vi "Catcher.vi"(0 "Catcher Position":i8) -> ()   [LabVIEW 2012]
uses:
  Robot Global Data.vi
  <vilib>/Rock Robotics/WPI/Joystick/WPI_JoystickGetSetRefNum.vi
panel:
  in  "Roller Speed Hold Low":dbl=-0.3
  out "High-Speed Toggle":bool
  in  "Bridge Position":dbl=2.8
  out "Joystick Control":bool
  in  "Joystick Speed Divider":dbl=2.0
  in  "Joystick Up Factor":dbl=1.5
  in  "Roller Speed Hold High":dbl=-0.3
  out "Button 11 Toggle":bool
  in  "Perimeter Threshold":dbl=1.1
  in  "Max Speeds":cluster{"Down Speed":dbl, "Up Speed":dbl}={"Down Speed"=0.45, "Up Speed"=-0.7}
  in  "PID gains":T1={"proportional gain (Kc)"=1.0, "integral time (Ti, min)"=0.0, "derivative time (Td, min)"=0.0} {"derivative time (Td, min)" format="%.3f"; "integral time (Ti, min)" format="%.3f"; "proportional gain (Kc)" format="%.3f"}
  out "Override":bool
  in  "Roller Speed Shoot":dbl=0.4
  in  "Dump Position":dbl=3.5
  out "Inside Perimeter":bool=TRUE
  in  "Catch Position":dbl=4.5
  in  "Rest Position":dbl=1.0
  out "Pot Voltage":dbl=1.0584093950000002
  # "0 - Hold Position\n1 - Catch\n2 - Dump\n4 - Bridge\n8 - Rest"
  # "4.5"
  # "0.8"
  # "0.35"
  # "3.5"
  # "-0.45"
  # "-0.6"
  # "2.8"
  # "-0.5"
  # "1"
  # "0.85"
  # "1"
  # "0"
  # "0"
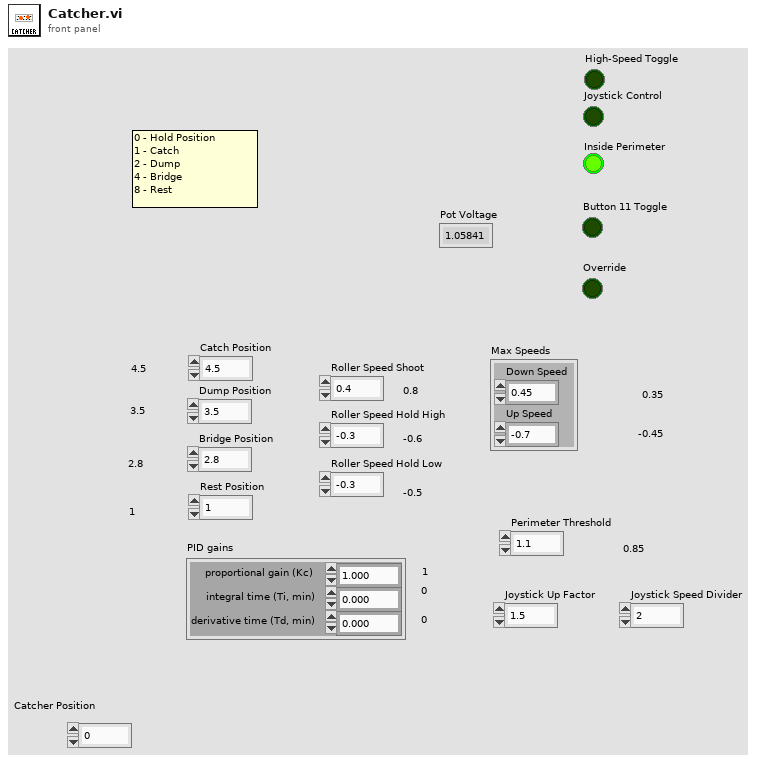
[diagram p1: front panel]
types:
  T1 = cluster{"proportional gain (Kc)":dbl, "integral time (Ti, min)":dbl, "derivative time (Td, min)":dbl}
  T2 = typedef "WPI_JoystickDevRef.ctl" = cluster{"Device":T3}
  T3 = typedef "WPI_JoystickDeviceEnum.ctl" = enum16{"USB 1", "USB 2", "USB 3", "USB 4", "Kinect 1", "Kinect 2"}
  T4 = typedef "WPI_JoystickButtonState.ctl" = cluster{"Button 1":bool, "Button 2":bool, "Button 3":bool, "Button 4":bool, "Button 5":bool, "Button 6":bool, "Button 7":bool, "Button 8":bool, "Button 9":bool, "Button 10":bool, "Button 11":bool, "Button 12":bool}
  T5 = cluster{"axis 1 (x)":dbl, "axis 2 (y)":dbl, "axis 3 (throttle)":dbl, "axis 4":dbl, "axis 5":dbl, "axis 6":dbl}
  T6 = typedef "WPI_AnalogChannelDevRef.ctl" = cluster{"DevStatus":errorcluster, "Analog Module":T7, "Analog Channel":T8}
  T7 = typedef "FPGA_TypedefAnalogModule.ctl" = enum16{"Analog Module 1", "Analog Module 2"}
  T8 = typedef "FPGA_AIChannel.ctl" = enum8{"AI 1", "AI 2", "AI 3", "AI 4", "AI 5", "AI 6", "AI 7", "AI 8", "Invalid"}
  T9 = typedef "WPI_MotorControlDeviceRef.ctl" = cluster{"DeviceStatus":errorcluster, "Type":enum16{"PWM", "CAN"}, "PWM":cluster{"Digital Module":T10, "PWM Channel":T11, "DeadBand":T12}, "CAN":cluster{"Device Number":u8, "Control Mode":T13, "Semaphore":T14, "Max Vout":dbl}, "Invert":bool, "TransformRef":T15, "InvTransformRef":T15}
  T10 = typedef "FPGA_TypedefDigitalModule.ctl" = enum16{"Digital Module 1", "Digital Module 2"}
  T11 = typedef "FPGA_DIOPWMChannel.ctl" = enum8{"PWM 1", "PWM 2", "PWM 3", "PWM 4", "PWM 5", "PWM 6", "PWM 7", "PWM 8", "PWM 9", "PWM 10", "Invalid"}
  T12 = typedef "WPI_PWMDeadband.ctl" = cluster{"Name":string, "maxPositivePwm":i32, "minPositivePwm":i32, "centerPwm":i32, "maxNegativePwm":i32, "minNegativePwm":i32, "angularRange":u16}
  T13 = typedef "WPI_CANJaguar_ControlMode.ctl" = enum8{"Percent VBus", "Current", "Speed", "Position", "Voltage"}
  T14 = typedef "Semaphore RefNum" = refnum<k1>
  T15 = typedef "WPI_PWMTransform_ConPane.ctl" = refnum<vi>
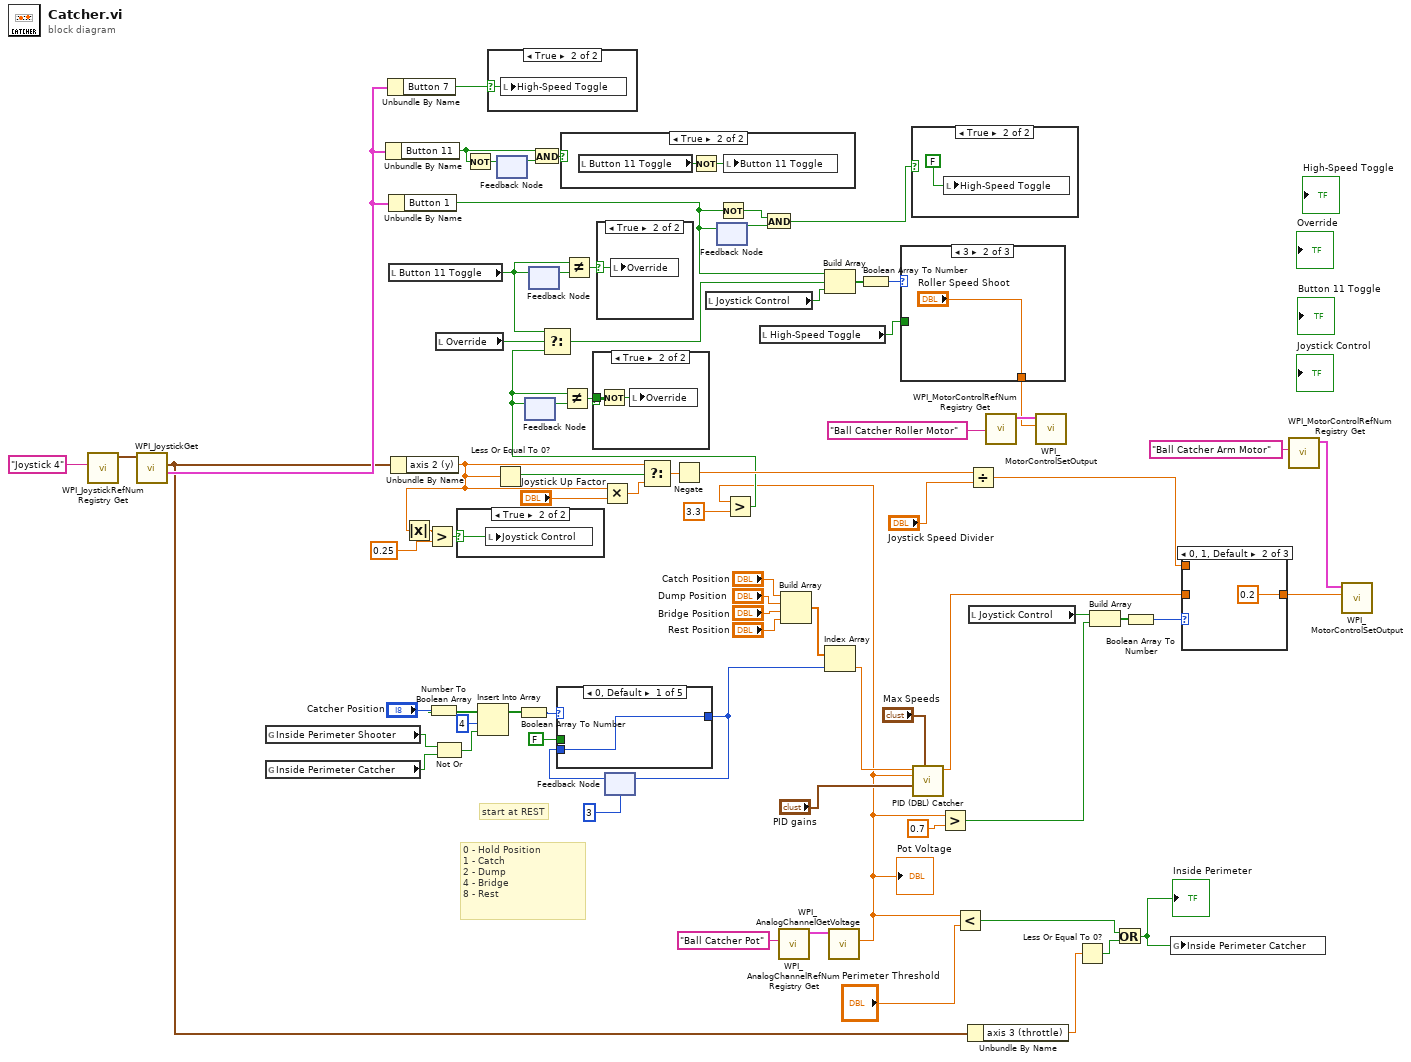
[diagram p0: block diagram]
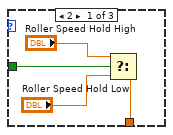
[diagram p6: hidden frame]
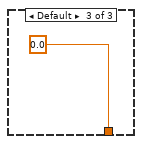
[diagram p7: hidden frame]
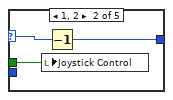
[diagram p12: hidden frame]
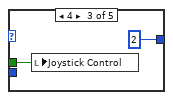
[diagram p13: hidden frame]
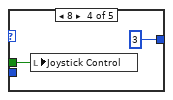
[diagram p14: hidden frame]
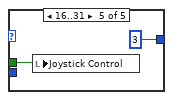
[diagram p15: hidden frame]
diagram:
  # "start at REST"
  # "0 - Hold Position\n1 - Catch\n2 - Dump\n4 - Bridge\n8 - Rest"
  n1 = call <vilib>:"WPI_JoystickRefNum Registry Get.vi"("refnum name"="Joystick 4") -> ("JoystickDevRef"=w70:T2)  [unwired: 9 in, 1 out]
  n2 = call <vilib>:"WPI_JoystickGet.vi"("JoystickDevRef"=w70) -> ("Buttons"=w16:T4, "Axes"=w9:T5)  [unwired: 4 in, 1 out]
  n3 = global read "Robot Global Data.vi" "Inside Perimeter Shooter"() -> (w42:bool)
  n4 = global read "Robot Global Data.vi" "Inside Perimeter Catcher"() -> (w41:bool)
  n5 = Unbundle By Name(w16) -> ("Button 11"=w50:bool)
  n6 = Unbundle By Name(w16) -> ("Button 7"=w15:bool)
  n7 = Unbundle By Name(w16) -> ("Button 1"=w14:bool)
  n8 = local read "Button 11 Toggle"() -> (w35:bool)
  n9 = Unbundle By Name(w9) -> ("axis 2 (y)"=w3:dbl)
  n10 = Absolute Value(x=w3) -> (abs(x)=w1:dbl)
  n11 = Greater?(x=w1, y=0.25 ("Joystick Threshold")) -> (0:w4:bool)
  n12 = Number To Boolean Array(number="Catcher Position") -> (Boolean array=w20:bool[])
  n13 = Not Or(1:w41, 2:w42) -> (0:w19:bool)
  n14 = local read "Override"() -> (w61:bool)
  n15 = case shown="True" w4 {
    selector: w4 -> [_ w78]
    frame False {
    }
    frame True {
      n16 = local write "Joystick Control"(w78) -> ()
    }
  }
  n17 = Not(x=w50) -> (.not. x?=w49:bool)
  n18 = Insert Into Array(array=w20, index=4, new element=w19) -> (w18:bool[])
  n19 = case shown="True" w15 {
    selector: w15 -> [_ w79]
    frame False {
    }
    frame True {
      n20 = local write "High-Speed Toggle"(w79) -> ()
    }
  }
  n21 = Less Or Equal To 0?(x=w3) -> (x <= 0?=w47:bool)
  n22 = feedback-in #1(w49) -> ()
  n23 = feedback #1() -> (w51:bool)  [unwired: 1 in]
  n24 = Boolean Array To Number(Boolean array=w18) -> (number=w63:u32)
  n25 = feedback #2() -> (w59:bool)  [unwired: 1 in]
  n26 = feedback #3() -> (w57:bool)  [unwired: 1 in]
  n27 = feedback-in #3(w35) -> ()
  n28 = And(x=w50, y=w51) -> (x .and. y?=w48:bool)
  n29 = case shown="True" w48 {
    frame False {
    }
    frame True {
      n30 = local read "Button 11 Toggle"() -> (w81:bool)
      n31 = Not(x=w81) -> (.not. x?=w80:bool)
      n32 = local write "Button 11 Toggle"(w80) -> ()
    }
  }
  n33 = Not Equal?(x=w35, y=w57) -> (x != y?=w58:bool)
  n34 = case shown="True" w58 {
    selector: w58 -> [_ w82]
    frame False {
    }
    frame True {
      n35 = local write "Override"(w82) -> ()
    }
  }
  n36 = Multiply(x=w3, y="Joystick Up Factor") -> (x*y=w46:dbl)
  n37 = feedback #4(u32 3) -> (w73:u32)
  n38 = case shown="0, Default" w63 {
    selector: w63 -> [_ w86 _ _ _]
    tunnel: w73 -> [w83 _ _ _ _]
    tunnel: [w83 w85 i8 2 3 u32 3] -> w43
    tunnel: FALSE ("Joystick Control") -> [_ w84 w87 w89 w91]
    frame 0, Default {
    }
    frame 1, 2 {
      n39 = local write "Joystick Control"(w84) -> ()
      n40 = Decrement(x=w86) -> (x-1=w85:u32)
    }
    frame 4 {
      n41 = local write "Joystick Control"(w87) -> ()
    }
    frame 8 {
      n42 = local write "Joystick Control"(w89) -> ()
    }
    frame 16..31 {
      n43 = local write "Joystick Control"(w91) -> ()
    }
  }
  n44 = feedback-in #4(w43) -> ()
  n45 = Select(t=w3, s=w47, f=w46) -> (s? t:f=w44:dbl)
  n46 = Negate(x=w44) -> (-x=w62:dbl)
  n47 = local read "Joystick Control"() -> (w22:bool)
  n48 = feedback-in #5(w14) -> ()
  n49 = feedback #5() -> (w12:bool)  [unwired: 1 in]
  n50 = Not(x=w14) -> (.not. x?=w13:bool)
  n51 = local read "High-Speed Toggle"() -> (w10:bool)
  n52 = And(x=w13, y=w12) -> (x .and. y?=w11:bool)
  n53 = call <vilib>:"WPI_AnalogChannelRefNum Registry Get.vi"("refnum name"="Ball Catcher Pot") -> ("AIDeviceRef"=w75:T6)  [unwired: 9 in, 1 out]
  n54 = Build Array("Catch Position", "Dump Position", "Bridge Position", "Rest Position") -> (w74:dbl[])
  n55 = Index Array(array=w74, index=w43) -> (element=w54:dbl)
  n56 = call <vilib>:"WPI_AnalogChannelGetVoltage.vi"("AIDeviceRef"=w75) -> ("Voltage"=w32:dbl)  [unwired: 8 in, 2 out]
  "Pot Voltage" <- w32
  n57 = Greater?(x=w32, y=3.3) -> (0:w60:bool)
  n58 = feedback-in #2(w60) -> ()
  n59 = Select(t=w35, s=w61, f=w60) -> (s? t:f=w30:bool)
  n60 = Not Equal?(x=w60, y=w59) -> (x != y?=w39:bool)
  n61 = case shown="True" w39 {
    tunnel: w39 -> [_ w94]
    frame False {
    }
    frame True {
      n62 = Not(x=w94) -> (.not. x?=w93:bool)
      n63 = local write "Override"(w93) -> ()
    }
  }
  n64 = Build Array(w14, w30, w22) -> (w38:bool[])
  n65 = Boolean Array To Number(Boolean array=w38) -> (number=w37:u32)
  n66 = case shown="3" w37 {
    tunnel: [w96 "Roller Speed Shoot" 0.0 ("f")] -> w36
    tunnel: w10 -> [w95 _ _]
    frame 2 {
      n67 = Select(t="Roller Speed Hold High", s=w95, f="Roller Speed Hold Low") -> (s? t:f=w96:dbl)
    }
    frame 3 {
    }
    frame Default {
    }
  }
  n68 = case shown="True" w11 {
    frame False {
    }
    frame True {
      n69 = local write "High-Speed Toggle"(FALSE) -> ()
    }
  }
  n70 = call "PID (DBL) Catcher.vi"("output range"="Max Speeds", "PID gains"="PID gains", "process variable"=w32, "setpoint"=w54) -> ("output"=w24:dbl)  [unwired: 6 in, 1 out]
  n71 = Greater?(x=w32, y=0.7) -> (0:w26:bool)
  n72 = Less?(x=w32, y="Perimeter Threshold") -> (x < y?=w6:bool)
  n73 = Divide(x=w62, y="Joystick Speed Divider") -> (x/y=w25:dbl)
  n74 = Unbundle By Name(w9) -> ("axis 3 (throttle)"=w8:dbl)
  n75 = local read "Joystick Control"() -> (w27:bool)
  n76 = call <vilib>:"WPI_MotorControlRefNum Registry Get.vi"("refnum name"="Ball Catcher Roller Motor") -> ("MotorControlDevRef"=w71:T9)  [unwired: 9 in, 1 out]
  n77 = call <vilib>:"WPI_MotorControlSetOutput.vi"("Output"=w36, "MotorControlDevRef"=w71) -> ()  [unwired: 7 in, 3 out]
  n78 = Less Or Equal To 0?(x=w8) -> (x <= 0?=w7:bool)
  n79 = Build Array(w27, w26) -> (w28:bool[])
  n80 = Or(x=w6, y=w7) -> (x .or. y?=w5:bool)
  "Inside Perimeter" <- w5
  n81 = Boolean Array To Number(Boolean array=w28) -> (number=w29:u32)
  n82 = global write "Robot Global Data.vi" "Inside Perimeter Catcher"(w5) -> ()
  n83 = case shown="0, 1, Default" w29 {
    tunnel: [w102 0.2 ("f") w104] -> w23
    tunnel: w24 -> [_ _ w104]
    tunnel: w25 -> [w102 _ _]
    frame 3 {
    }
    frame 0, 1, Default {
    }
    frame 2 {
    }
  }
  n84 = call <vilib>:"WPI_MotorControlRefNum Registry Get.vi"("refnum name"="Ball Catcher Arm Motor") -> ("MotorControlDevRef"=w77:T9)  [unwired: 9 in, 1 out]
  n85 = call <vilib>:"WPI_MotorControlSetOutput.vi"("Output"=w23, "MotorControlDevRef"=w77) -> ()  [unwired: 7 in, 3 out]
